vi "tm488_attachbuffersnap_wVision.vi"() -> ()   [LabVIEW 2019]
panel:
  out "Image":T1(plugin-control)
  in  "Play":bool
  in  "Acquire":bool
  out "Current Frame Index":i32=-1
  in  "Frames to Capture":i32=100
  out "Camera Serial":string
  out "Camera Model":string
  out "Camera Version":string
  out "Total Frames":i32
  out "error out":errorcluster {"code" format="%.0x"}
  in  "quit":bool
  # "This is an example of how to attach\nyour own data buffers to the capture\nlibrary."
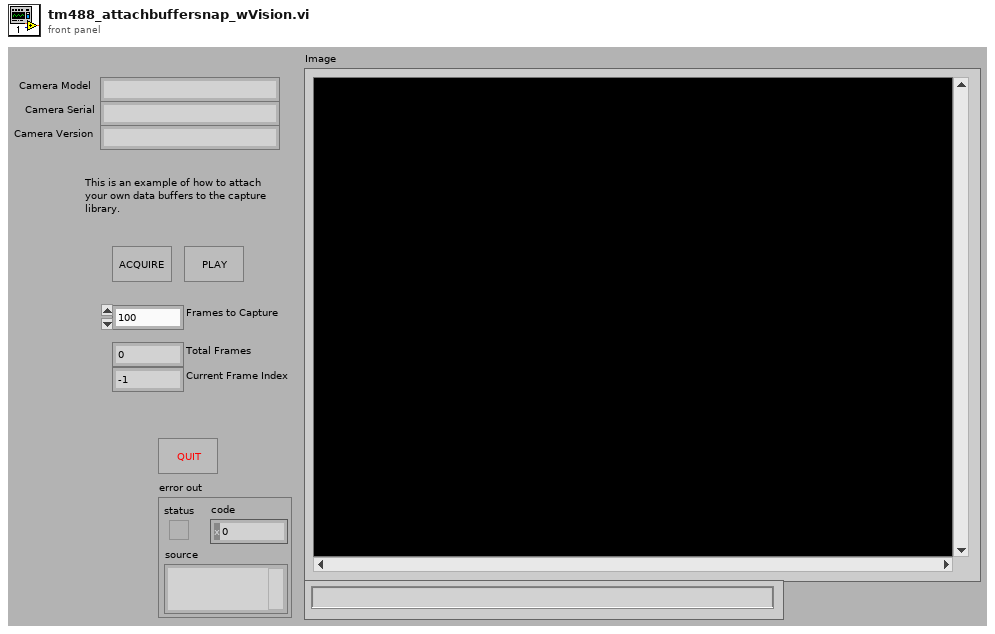
[diagram p1: front panel]
types:
  T1 = typedef "IMAQ Image.ctl" = refnum<image>
  T2 = enum32{"Map Pixel Pointer", "Unmap Pixel Pointer", "Get Pixels Infos"}
  T3 = cluster{"Model":string, "Camera ID":string, "Firmware":string}
  T4 = typedef "Image Type" = u32
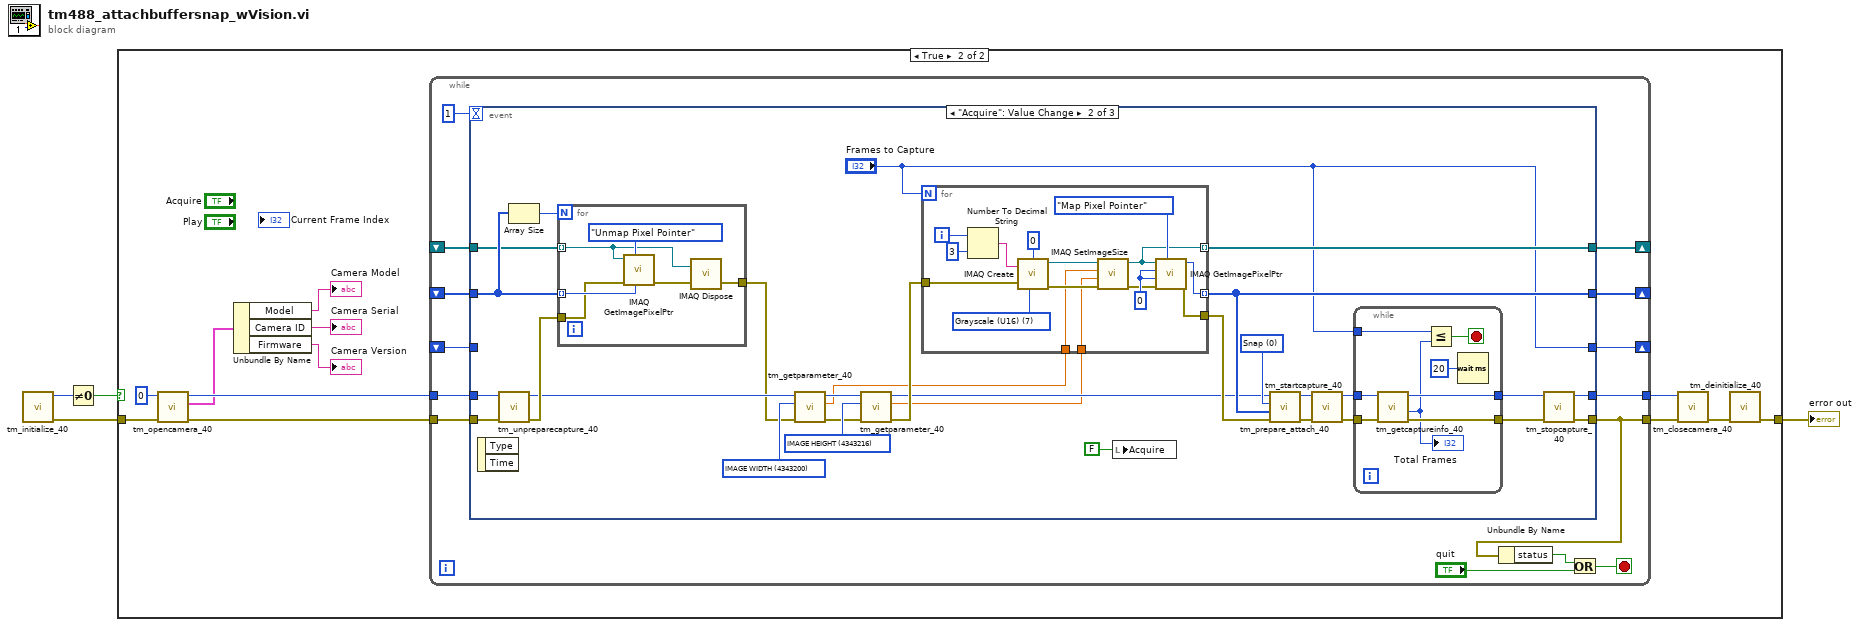
[diagram p0: block diagram]
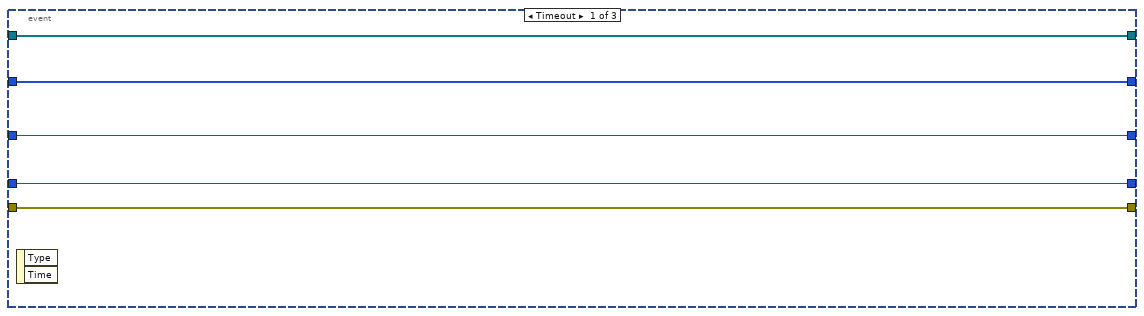
[diagram p3: hidden frame]
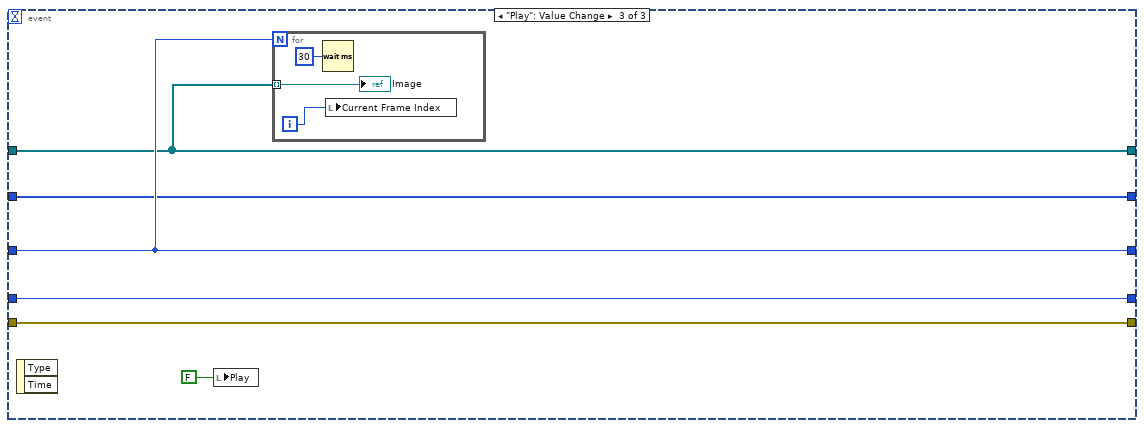
[diagram p4: hidden frame]
diagram:
  n1 = call <userlib>:"tm_initialize_40.vi"() -> ("error out"=w1:errorcluster, "Number Of Cameras"=w2:u32)  [unwired: 8 in, 2 out]
  n2 = Not Equal To 0?(x=w2) -> (x != 0?=w4:bool)
  n3 = case shown="True" w4 {
    tunnel: [w5 w14] -> w3
    tunnel: w1 -> [w5 w17]
    frame False {
    }
    frame True {
      n4 = call <userlib>:"tm_opencamera_40.vi"("error in (no error)"=w17, "Camera Index"=u32 0) -> ("error out"=w9:errorcluster, "Camera Details"=w10:T3, "Handle out"=w13:u32)  [unwired: 7 in]
      n5 = Unbundle By Name(w10) -> ("Model"=→"Camera Model":string, "Camera ID"=→"Camera Serial":string, "Firmware"=→"Camera Version":string)
      n6 = while {
        tunnel: [w26] -> w12
        tunnel: [w31] -> w11
        tunnel: w13 -> [w29]
        tunnel: w9 -> [w28]
        shift-right: [w23] -> _
        shift-left: _ -> [w27]
        shift-right: [w21] -> _
        shift-left: _ -> [w19]
        shift-right: [w20] -> _
        shift-left: _ -> [w18]
        stop <- w22 stop-if-true
        n7 = event shown="[1] \"Acquire\": Value Change" {
          selector: _ -> [_ _ _]
          dyn-events: _ -> [_ _ _]
          timeout: 1 -> [_ _ _]
          tunnel: [w35 w64 w98] -> w31
          tunnel: [w36 w65 w97] -> w26
          tunnel: w28 -> [w36 w63 w97]
          tunnel: w29 -> [w35 w62 w98]
          tunnel: [w34 "Frames to Capture" w102] -> w23
          tunnel: w27 -> [w34 _ w102]
          tunnel: [w32 w57 w99] -> w21
          tunnel: [w33 w58 w100] -> w20
          tunnel: w19 -> [w32 w56 w99]
          tunnel: w18 -> [w33 w54 w100]
          event Timeout {
            n8 = event-data() -> ()  [unwired: 1 in, 2 out]
          }
          event "Acquire": Value Change {
            w51 = u32 4343216 items=["SENSOR MODE"=4212128, "READOUT SPEED"=4211872, "READOUT DIRECTION"=4211904, "TRIGGER GLOBAL EXPOSURE"=2049680, "TRIGGER DELAY"=1066480, "INTERNAL TRIGGER HANDLING"=1066496, "SENSOR TEMPERATURE"=2115232, "SENSOR COOLER STATUS"=2115280, "EXPOSURE TIME"=2049184, "DEFECT CORRECT MODE"=4670368, "HOT PIXEL CORRECT LEVEL"=4670400, "BINNING"=4215968, "TIMING READOUT TIME"=4223904, "INTERNAL FRAME RATE"=4225952, "INTERNAL FRAME INTERVAL"=4225968, "INTERNAL LINE SPEED"=4226000, "INTERNAL LINE INTERVAL"=4226016, "IMAGE WIDTH"=4343200, "IMAGE HEIGHT"=4343216, "IMAGE ROWBYTES"=4343232, "IMAGE FRAMEBYTES"=4343248, "IMAGE PIXEL TYPE"=4343296, "NUMBER OF OUTPUT TRIGGER CONNECTOR"=1852320, "OUTPUT TRIGGER SOURCE[0]"=1852576, "OUTPUT TRIGGER SOURCE[1]"=1852832, "OUTPUT TRIGGER SOURCE[2]"=1853088, "OUTPUT TRIGGER POLARITY[0]"=1852592, "OUTPUT TRIGGER POLARITY[1]"=1852848, "OUTPUT TRIGGER POLARITY[2]"=1853104, "OUTPUT TRIGGER ACTIVE[0]"=1852608, "OUTPUT TRIGGER ACTIVE[1]"=1852864, "OUTPUT TRIGGER ACTIVE[2]"=1853120, "OUTPUT TRIGGER DELAY[0]"=1852624, "OUTPUT TRIGGER DELAY[1]"=1852880, "OUTPUT TRIGGER DELAY[2]"=1853136, "OUTPUT TRIGGER PERIOD[0]"=1852640, "OUTPUT TRIGGER PERIOD[1]"=1852896, "OUTPUT TRIGGER PERIOD[2]"=1853152, "OUTPUT TRIGGER KIND[0]"=1852656, "OUTPUT TRIGGER KIND[1]"=1852912, "OUTPUT TRIGGER KIND[2]"=1853168, "OUTPUT TRIGGER BASE SENSOR[0]"=1852672, "OUTPUT TRIGGER BASE SENSOR[1]"=1852928, "OUTPUT TRIGGER BASE SENSOR[2]"=1853184, "OUTPUT TRIGGER PRE HSYNC COUNT"=1852704] ("Parameter")
            w52 = u32 4343200 items=["SENSOR MODE"=4212128, "READOUT SPEED"=4211872, "READOUT DIRECTION"=4211904, "TRIGGER GLOBAL EXPOSURE"=2049680, "TRIGGER DELAY"=1066480, "INTERNAL TRIGGER HANDLING"=1066496, "SENSOR TEMPERATURE"=2115232, "SENSOR COOLER STATUS"=2115280, "EXPOSURE TIME"=2049184, "DEFECT CORRECT MODE"=4670368, "HOT PIXEL CORRECT LEVEL"=4670400, "BINNING"=4215968, "TIMING READOUT TIME"=4223904, "INTERNAL FRAME RATE"=4225952, "INTERNAL FRAME INTERVAL"=4225968, "INTERNAL LINE SPEED"=4226000, "INTERNAL LINE INTERVAL"=4226016, "IMAGE WIDTH"=4343200, "IMAGE HEIGHT"=4343216, "IMAGE ROWBYTES"=4343232, "IMAGE FRAMEBYTES"=4343248, "IMAGE PIXEL TYPE"=4343296, "NUMBER OF OUTPUT TRIGGER CONNECTOR"=1852320, "OUTPUT TRIGGER SOURCE[0]"=1852576, "OUTPUT TRIGGER SOURCE[1]"=1852832, "OUTPUT TRIGGER SOURCE[2]"=1853088, "OUTPUT TRIGGER POLARITY[0]"=1852592, "OUTPUT TRIGGER POLARITY[1]"=1852848, "OUTPUT TRIGGER POLARITY[2]"=1853104, "OUTPUT TRIGGER ACTIVE[0]"=1852608, "OUTPUT TRIGGER ACTIVE[1]"=1852864, "OUTPUT TRIGGER ACTIVE[2]"=1853120, "OUTPUT TRIGGER DELAY[0]"=1852624, "OUTPUT TRIGGER DELAY[1]"=1852880, "OUTPUT TRIGGER DELAY[2]"=1853136, "OUTPUT TRIGGER PERIOD[0]"=1852640, "OUTPUT TRIGGER PERIOD[1]"=1852896, "OUTPUT TRIGGER PERIOD[2]"=1853152, "OUTPUT TRIGGER KIND[0]"=1852656, "OUTPUT TRIGGER KIND[1]"=1852912, "OUTPUT TRIGGER KIND[2]"=1853168, "OUTPUT TRIGGER BASE SENSOR[0]"=1852672, "OUTPUT TRIGGER BASE SENSOR[1]"=1852928, "OUTPUT TRIGGER BASE SENSOR[2]"=1853184, "OUTPUT TRIGGER PRE HSYNC COUNT"=1852704] ("Parameter")
            w61 = 0 items=["Snap", "Sequence"] ("Capture mode")
            n9 = event-data() -> ()  [unwired: 1 in, 2 out]
            n10 = call <userlib>:"tm_unpreparecapture_40.vi"("error in (no error)"=w63, "Handle in"=w62) -> ("error out"=w50:errorcluster, "Handle out"=w49:u32)  [unwired: 8 in]
            n11 = Array Size(array=w56) -> (size(s)=w55:i32)
            n12 = for {
              N: w55 -> [_]
              tunnel: w56 -> [w80] mode=indexing
              tunnel: w54 -> [w78] mode=indexing
              tunnel: w50 -> [w76]
              tunnel: [w75] -> w46
              n13 = call "IMAQ GetImagePixelPtr"("Pixel Pointer in"=w80, "Function"=T2."Unmap Pixel Pointer", "error in (no error)"=w76, "Image"=w78) -> ("error out"=w77:errorcluster)  [unwired: 2 in, 5 out]
              n14 = call "IMAQ Dispose"("Image"=w78, "error in (no error)"=w77) -> ("error out"=w75:errorcluster)  [unwired: 4 in]
            }
            n15 = call <userlib>:"tm_getparameter_40.vi"("error in (no error)"=w46, "Parameter"=w52, "Handle in"=w49) -> ("error out"=w48:errorcluster, "Value out"=w43:dbl, "Handle out"=w47:u32)  [unwired: 6 in]
            n16 = call <userlib>:"tm_getparameter_40.vi"("error in (no error)"=w48, "Parameter"=w51, "Handle in"=w47) -> ("error out"=w45:errorcluster, "Value out"=w42:dbl, "Handle out"=w44:u32)  [unwired: 6 in]
            n17 = for {
              N: "Frames to Capture" -> [_]
              tunnel: [w85] -> w58 mode=indexing
              tunnel: [w90] -> w57 mode=indexing
              tunnel: w45 -> [w84]
              tunnel: [w83] -> w53
              tunnel: w43 -> [w82]
              tunnel: w42 -> [w81]
              i -> [w96]
              w87 = T4 7 items=["Grayscale (U8)", "Grayscale (I16)", "Grayscale (SGL)", "Complex (CSG)", "RGB (U32)", "HSL (U32)", "RGB (U64)", "Grayscale (U16)"] ("Image Type")
              w91 = 0 ("X Coordinate")
              n18 = Number To Decimal String(number=w96, width (-)=i16 3) -> (decimal integer string=w94:string)
              n19 = call "IMAQ Create"("Border Size"=0, "Image Name"=w94, "Image Type"=w87, "error in (no error)"=w84) -> ("New Image"=w89:T1, "error out"=w88:errorcluster)  [unwired: 1 in]
              n20 = call "IMAQ SetImageSize"("error in (no error)"=w88, "Y Resolution"=w81, "X Resolution"=w82, "Image"=w89) -> ("error out"=w86:errorcluster, "Image Out"=w85:T1)  [unwired: 1 in]
              n21 = call "IMAQ GetImagePixelPtr"("Function"=T2."Map Pixel Pointer", "error in (no error)"=w86, "Y Coordinate"=w91, "X Coordinate"=w91, "Image"=w85) -> ("error out"=w83:errorcluster, "Pixel Pointer out"=w90:u64)  [unwired: 1 in, 4 out]
            }
            n22 = local write "Acquire"(FALSE) -> ()
            n23 = call <userlib>:"tm_prepare_attach_40.vi"("error in (no error)"=w53, "buffers"=w57, "Capture mode"=w61, "Handle in"=w44) -> ("error out"=w59:errorcluster, "Handle out"=w60:u32)  [unwired: 6 in]
            n24 = call <userlib>:"tm_startcapture_40.vi"("error in (no error)"=w59, "Handle in"=w60) -> ("error out"=w41:errorcluster, "Handle out"=w40:u32)  [unwired: 8 in]
            n25 = while {
              tunnel: w41 -> [w74]
              tunnel: w40 -> [w73]
              tunnel: [w72] -> w38
              tunnel: [w71] -> w39
              tunnel: "Frames to Capture" -> [w70]
              stop <- w68 stop-if-true
              n26 = call <userlib>:"tm_getcaptureinfo_40.vi"("error in (no error)"=w74, "Handle in"=w73) -> ("error out"=w71:errorcluster, "Frame Count"=w69:i32, "Handle out"=w72:u32)  [unwired: 6 in, 1 out]
              "Total Frames" <- w69
              n27 = Less Or Equal?(x=w70, y=w69) -> (x <= y?=w68:bool)
              n28 = Wait (ms)(milliseconds to wait=u32 20) -> ()  [unwired: 1 out]
            }
            n29 = call <userlib>:"tm_stopcapture_40.vi"("error in (no error)"=w39, "Handle in"=w38) -> ("error out"=w65:errorcluster, "Handle out"=w64:u32)  [unwired: 8 in]
          }
          event "Play": Value Change {
            n30 = event-data() -> ()  [unwired: 1 in, 2 out]
            n31 = local write "Play"(FALSE) -> ()
            n32 = for {
              N: w102 -> [_]
              tunnel: w100 -> [w105] mode=indexing
              i -> [w103]
              n33 = Wait (ms)(milliseconds to wait=u32 30) -> ()  [unwired: 1 out]
              n34 = local write "Current Frame Index"(w103) -> ()
              "Image" <- w105
            }
          }
        }
        n35 = Unbundle By Name(w26) -> ("status"=w25:bool)
        n36 = Or(x=w25, y="quit") -> (x .or. y?=w22:bool)
      }
      n37 = call <userlib>:"tm_closecamera_40.vi"("error in (no error)"=w12, "Handle in"=w11) -> ("error out"=w15:errorcluster)  [unwired: 9 in]
      n38 = call <userlib>:"tm_deinitialize_40.vi"("error in (no error)"=w15) -> ("error out"=w14:errorcluster)  [unwired: 10 in]
    }
  }
  "error out" <- w3
